vi "运维调试_总氮.vi"() -> ()   [LabVIEW 2016, in "斯坦道总氮.lvlib"]
uses:
  <vilib>/Utility/miscctls.llb/LVPointTypeDef.ctl
  <vilib>/Utility/config.llb/NI_LVConfig.lvlib
  <vilib>/ptbypt/NI_PtbyPt.lvlib
panel:
  in  "模块启用":bool
  in  "串口设置":bool
  in  "备用系数一键写入":bool
  in  "公式一键写入":bool
  in  "流程路径":path=path "C:/Users/STD/Documents/斯坦道流程文件/流程.xml"
  in  "总磷总氮曲线模型":cluster{"X^2":dbl, "X":dbl, "B":dbl}(xcontrol)
  out "字符串 2":string
  in  "质控参数设置":bool
  in  "自动测试量程配置":T1
  out "温度2":sgl
  out "温度1":sgl
  out "ADC":sgl
  out "固件版本号":string
  in  "数组":string[](array[string])
  in  "备用系数写入":bool
  in  "备用系数读取":bool
  in  "备用系数":T2
  in  "量程切换阈值写入":bool
  in  "量程切换阈值读取":bool
  in  "量程切换阈值":cluster{"阈值":dbl, "标液浓度":dbl}
  in  "参数下拉列表":enum16{"总磷", "总氮"}(ring)=enum."总氮"
  in  "量程下拉列表":enum16{"低量程", "高量程"}(ring)
  in  "测量模式下拉列表":enum16{"水样测量", "空白核查", "跨度核查", "标样核查", "加标回收"}(ring)
  in  "公式":cluster{"X^2":dbl, "X":dbl, "b":dbl}
  in  "写公式":bool
  in  "读公式":bool
  in  "返回":bool
  in  "设置":bool
  out "序列号":string="序列号"
  out "测量数据":T3(xcontrol)
  out "集成报警信息":string
  out "定时启动":bool
  out "总磷总氮运行状态":T4(xcontrol)
  in  "停止":bool
  in  "手动启动":bool
  in  "单步测试":bool
  in  "总磷氨氮调试":u16[](xcontrol)
  out "F3":sgl format="%#.6f"
  out "F2":sgl format="%#.6f"
  out "F1":sgl format="%#.6f"
  out "F0":sgl format="%#.6f"
  out "多列列表框":i32(listbox)
  # "参数设置"
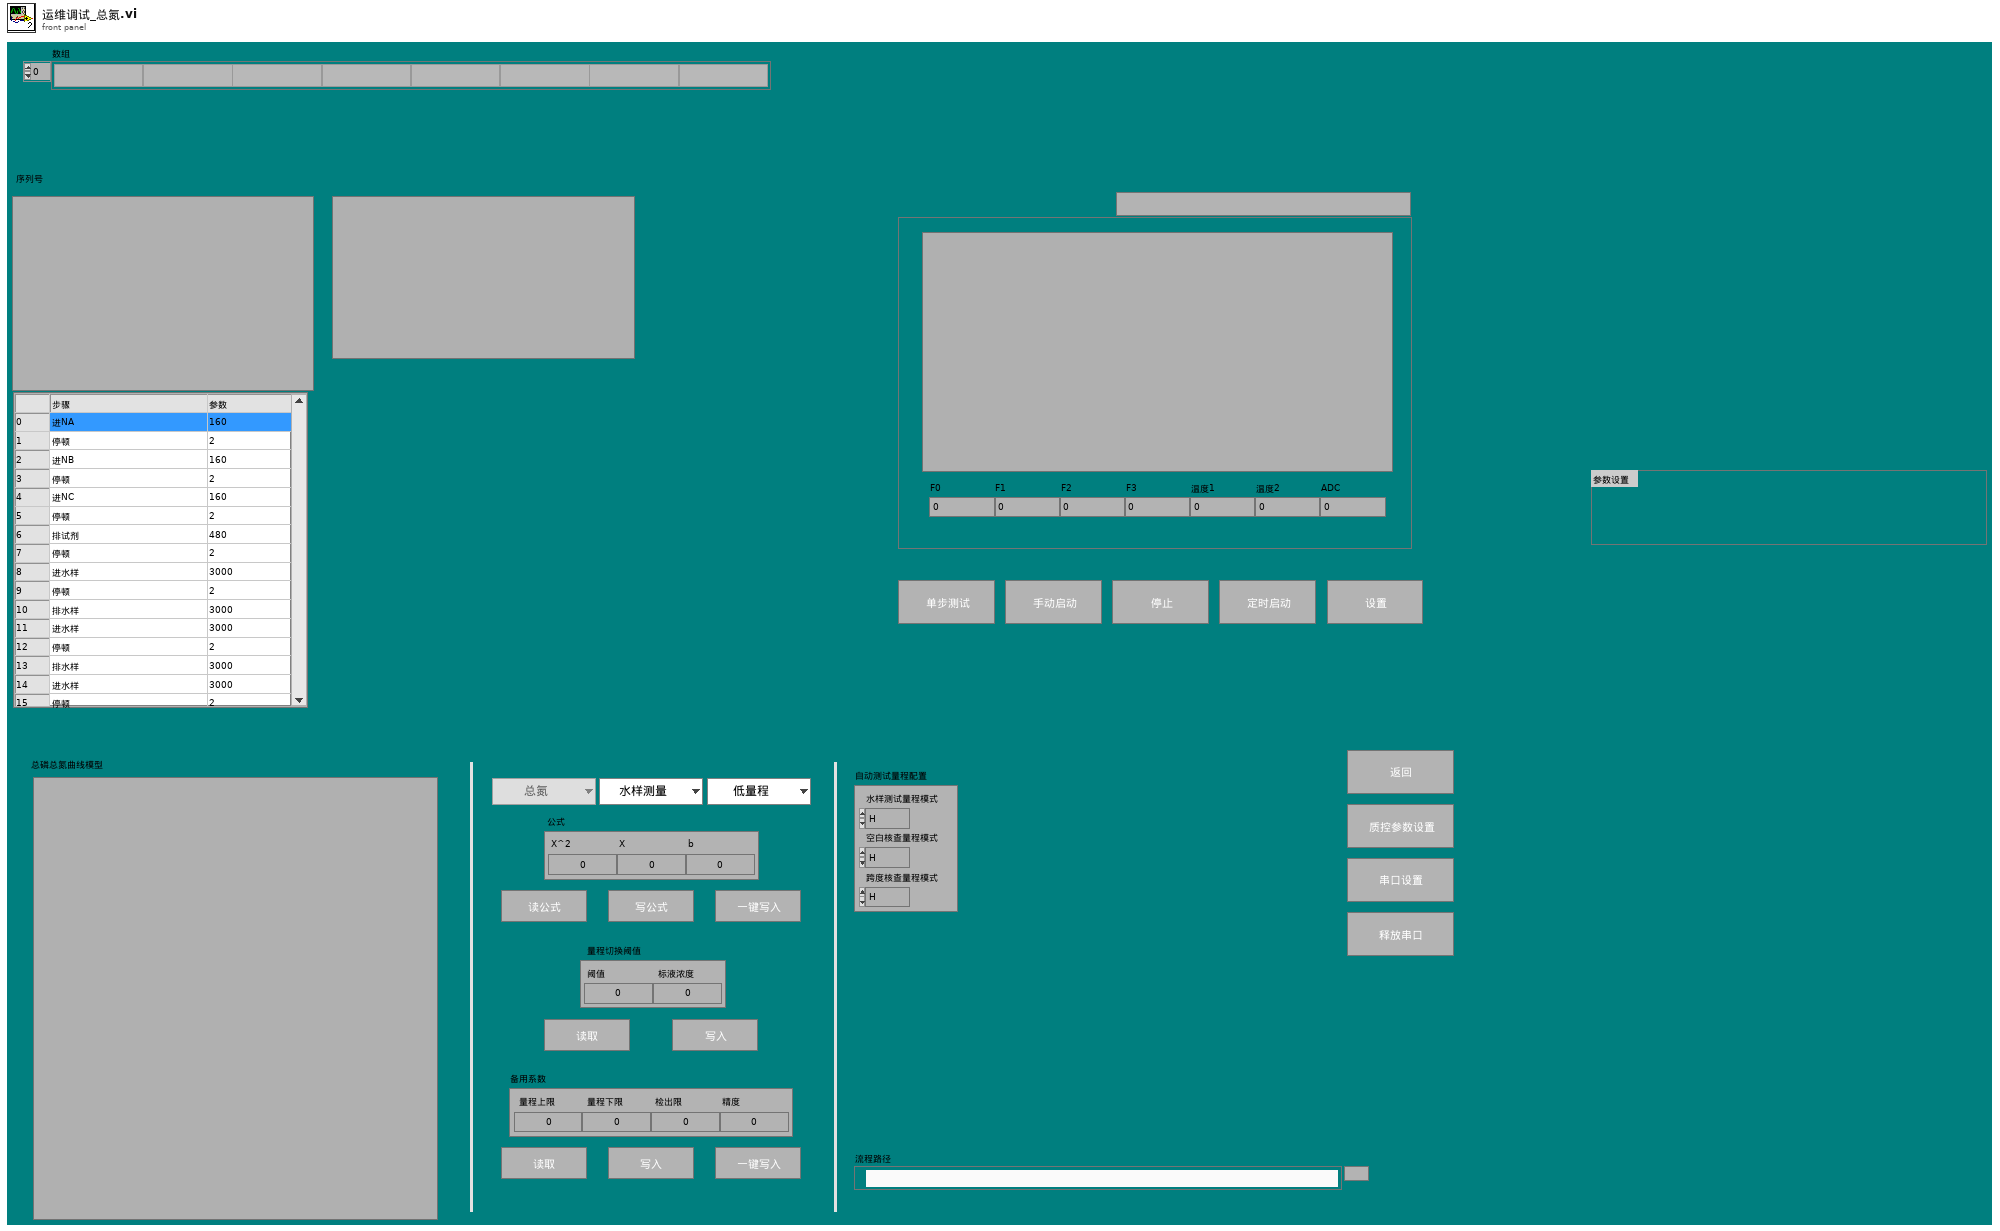
[diagram p1: front panel]
types:
  T1 = cluster{"水样测试量程模式":enum16{"H", "L", "AUTO"}, "空白核查量程模式":enum16{"H", "L", "AUTO"}, "跨度核查量程模式":enum16{"H", "L", "AUTO"}}
  T2 = cluster{"量程上限":dbl, "量程下限":dbl, "检出限":dbl, "精度":dbl}
  T3 = cluster{"flowid":u16, "测量精度":u16, "测量数据区":cluster{"因子编码":u32, "单位":u16, "标样参考值":sgl, "水样数据时间":timestamp, "水样实测值":sgl, "水样数据标识":string, "标样数据时间":timestamp, "标样实测值":sgl, "标样数据标识":string, "空白数据时间":timestamp, "空白实测值":sgl, "空白数据标识":string, "零点核查数据时间":timestamp, "零点核查实测值":sgl, "零点核查数据标识":string, "跨度核查数据时间":timestamp, "跨度核查实测值":sgl, "跨度核查数据标识":string, "加标回收数据时间":timestamp, "加标回收实测值":sgl, "加标回收数据标识":string, "平行样数据时间":timestamp, "平行样实测值":sgl, "平行样数据标识":string, "F0":sgl, "F1":sgl, "F2":sgl, "F3":sgl, "F4":sgl, "F5":sgl, "F6":sgl, "F7":sgl, "温度":sgl, "湿度":sgl, "X值":sgl}}
  T4 = cluster{"系统时间":timestamp, "工作状态":enum16{"空闲", "水样测试", "标样核查", "零点核查", "跨度核查", "空白测试", "平行样测试", "加标回收", "空白校准", "标样校准", "初始化（清洗）"}, "测量模式":enum16{"待机", "连续模式", "周期模式", "定点模式", "受控模式", "手动模式"}, "告警代码":enum16{"无告警", "缺试剂告警", "缺水样告警", "缺蒸馏水告警", "缺标液告警", "仪表漏液告警", "标定异常告警", "超量程告警", "加热异常", "低试剂预警", "超上限告警", "超下限告警", "仪表内部其他异常", "滴定异常告警", "电极异常告警", "量程切换告警", "参数设置告警", "PH电极电位异常", "电导率电极异常", "浊度光度异常", "溶解氧电极异常", "溶解氧光强异常", "温度异常告警", "PH异常告警", "溶解氧异常告警", "电导率异常告警", "浊度异常告警", "叶绿素异常告警", "藻密度异常告警", "蓝绿藻异常告警", "ORP异常告警", "氨氮异常告警", "清洁刷异常告警", "SD卡异常告警", "蓝牙异常告警", "Wifi异常告警", "流程异常告警"}, "故障代码":enum16{"无故障", "电机故障", "温度故障", "通讯故障", "滴定故障"}, "日志代码":u16, "软件版本":u16, "F0":sgl, "F1":sgl, "F2":sgl, "F3":sgl, "T":sgl, "H":sgl, "id":u16, "flowid":u16, "量程":u16, "总磷控温温度1":sgl, "营养盐控温温度2":sgl, "ADC":sgl}
  T5 = cluster{"控制命令":enum16{"启动测量", "标样核查", "零点核查", "跨度核查", "空白测试", "平行样测试", "加标回收", "空白校准", "标样校准", "初始化（清洗）", "停止测试", "仪器重启", "校时", "模式设置", "测量间隔设置"}, "周期设置类型":enum16{"定点启动", "间隔启动"}, "定时功能启用":bool, "定时间隔":dbl, "24H周期设置":bool[]}
  T6 = enum16{"启动测量", "标样核查", "零点核查", "跨度核查", "空白测试", "平行样测试", "加标回收", "空白校准", "标样校准", "初始化（清洗）", "停止测试", "仪器重启", "校时", "模式设置", "测量间隔设置"}
  T7 = enum32{"Bad", "Idle", "Run top level", "Running"}
  T8 = typedef "LVDateTimeRec.ctl" = cluster{"秒数的小数部分":dbl, "秒":i32, "分":i32, "时":i32, "日":i32, "月":i32, "年":i32, "天数（周）":i32, "天数（年）":i32, "DST":i32}
  T9 = typedef "LVPointTypeDef.ctl" = cluster{"Horizontal":i16, "Vertical":i16}
  T10 = cluster{"因子编码":u32, "单位":u16, "标样参考值":sgl, "水样数据时间":timestamp, "水样实测值":sgl, "水样数据标识":string, "标样数据时间":timestamp, "标样实测值":sgl, "标样数据标识":string, "空白数据时间":timestamp, "空白实测值":sgl, "空白数据标识":string, "零点核查数据时间":timestamp, "零点核查实测值":sgl, "零点核查数据标识":string, "跨度核查数据时间":timestamp, "跨度核查实测值":sgl, "跨度核查数据标识":string, "加标回收数据时间":timestamp, "加标回收实测值":sgl, "加标回收数据标识":string, "平行样数据时间":timestamp, "平行样实测值":sgl, "平行样数据标识":string, "F0":sgl, "F1":sgl, "F2":sgl, "F3":sgl, "F4":sgl, "F5":sgl, "F6":sgl, "F7":sgl, "温度":sgl, "湿度":sgl, "X值":sgl}
  T11 = enum16{"空闲", "水样测试", "标样核查", "零点核查", "跨度核查", "空白测试", "平行样测试", "加标回收", "空白校准", "标样校准", "初始化（清洗）"}
  T12 = typedef "NI_LVConfig.lvlib/Config Data RefNum.ctl" = refnum<k1>
  T13 = cluster{"启动模式":enum16{"跨度核查", "水样测量", "空白核查", "标样核查", "加标回收"}, "启动参数":u16, "量程":enum16{"低量程", "高量程"}}
  T14 = cluster{"时间标识":timestamp, "设备":string, "日志信息":string, "流程参数":string}
  T15 = cluster{"时间标识":timestamp, "设备":string, "日志信息":string}
  T16 = enum16{"无告警", "缺试剂告警", "缺水样告警", "缺蒸馏水告警", "缺标液告警", "仪表漏液告警", "标定异常告警", "超量程告警", "加热异常", "低试剂预警", "超上限告警", "超下限告警", "仪表内部其他异常", "滴定异常告警", "电极异常告警", "量程切换告警", "参数设置告警", "PH电极电位异常", "电导率电极异常", "浊度光度异常", "溶解氧电极异常", "溶解氧光强异常", "温度异常告警", "PH异常告警", "溶解氧异常告警", "电导率异常告警", "浊度异常告警", "叶绿素异常告警", "藻密度异常告警", "蓝绿藻异常告警", "ORP异常告警", "氨氮异常告警", "清洁刷异常告警", "SD卡异常告警", "蓝牙异常告警", "Wifi异常告警", "流程异常告警"}
  T17 = typedef "LVRowAndColumnUnsignedTypeDef.ctl" = cluster{"Row":u32, "Column":u32}
  T18 = cluster{"站号":u16, "量程切换":enum32{"H", "L", "AUTO"}, "控制命令":enum16{"启动测量", "标样核查", "零点核查", "跨度核查", "空白测试", "平行样测试", "加标回收", "空白校准", "标样校准", "初始化（清洗）", "停止测试", "仪器重启", "校时", "模式设置", "测量间隔设置"}, "模式设置":enum16{"待机", "连续模式", "周期模式", "定点模式", "受控模式", "手动模式"}, "测量间隔":u16}
  T19 = cluster{"跨度值":dbl, "零点标准液浓度":dbl, "跨度标准液浓度":dbl, "标准液标准浓度":dbl}
  T20 = cluster{"确定":bool, "跨度值":dbl, "零点标准液浓度":dbl, "跨度标准液浓度":dbl, "标准液标准浓度":dbl}
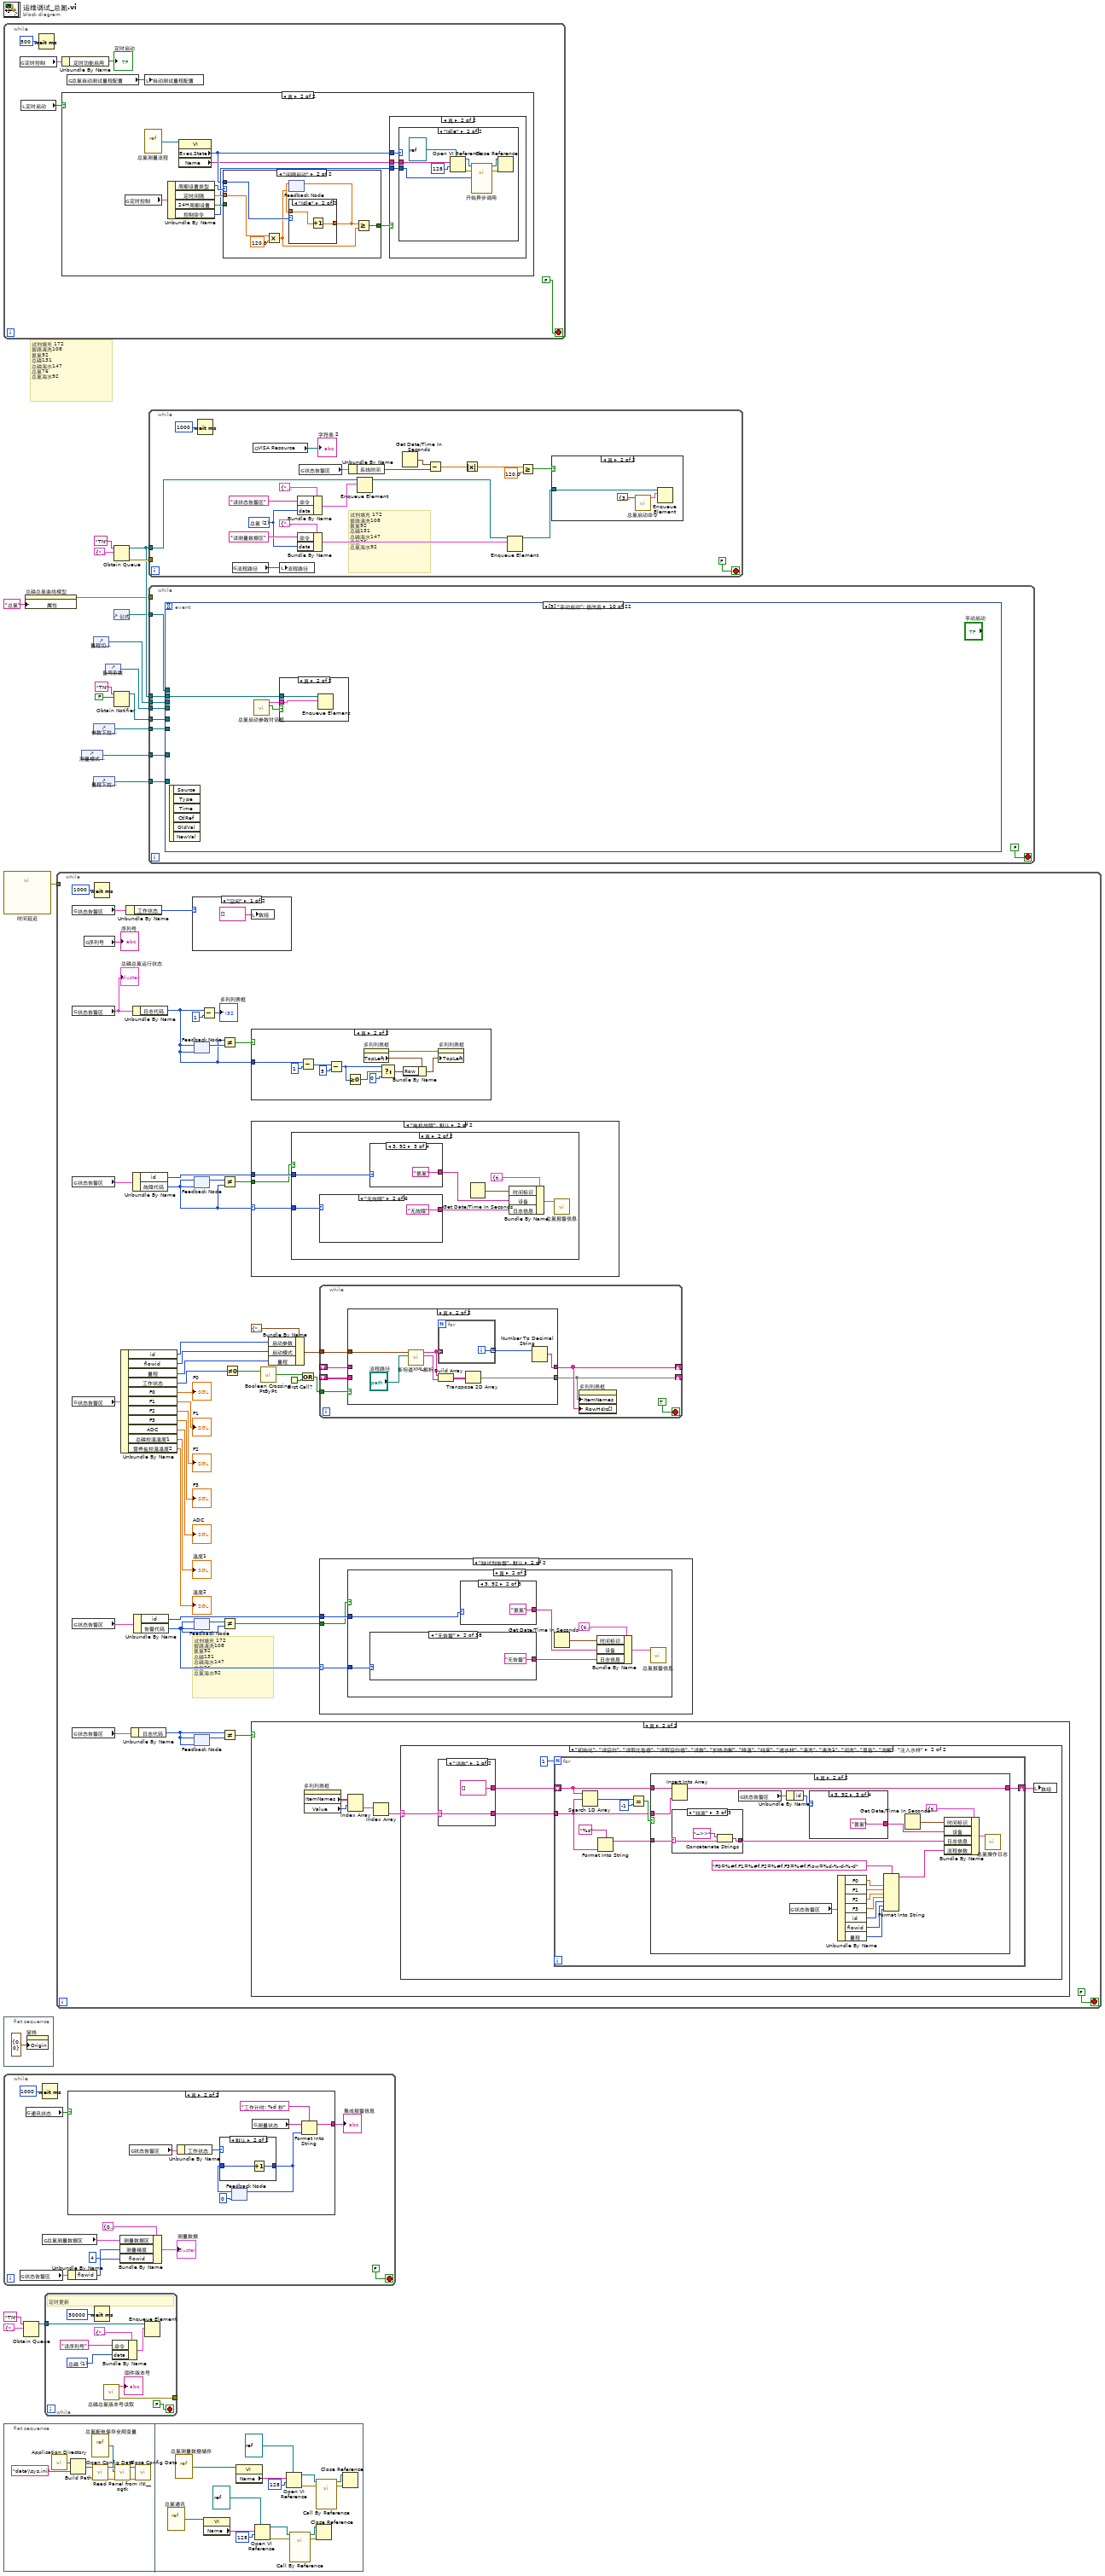
[diagram p0: block diagram]
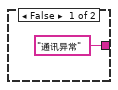
[diagram p2: hidden frame]
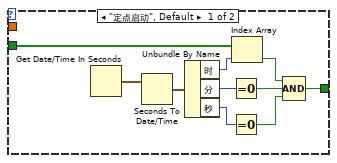
[diagram p7: hidden frame]
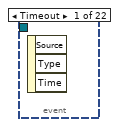
[diagram p9: hidden frame]
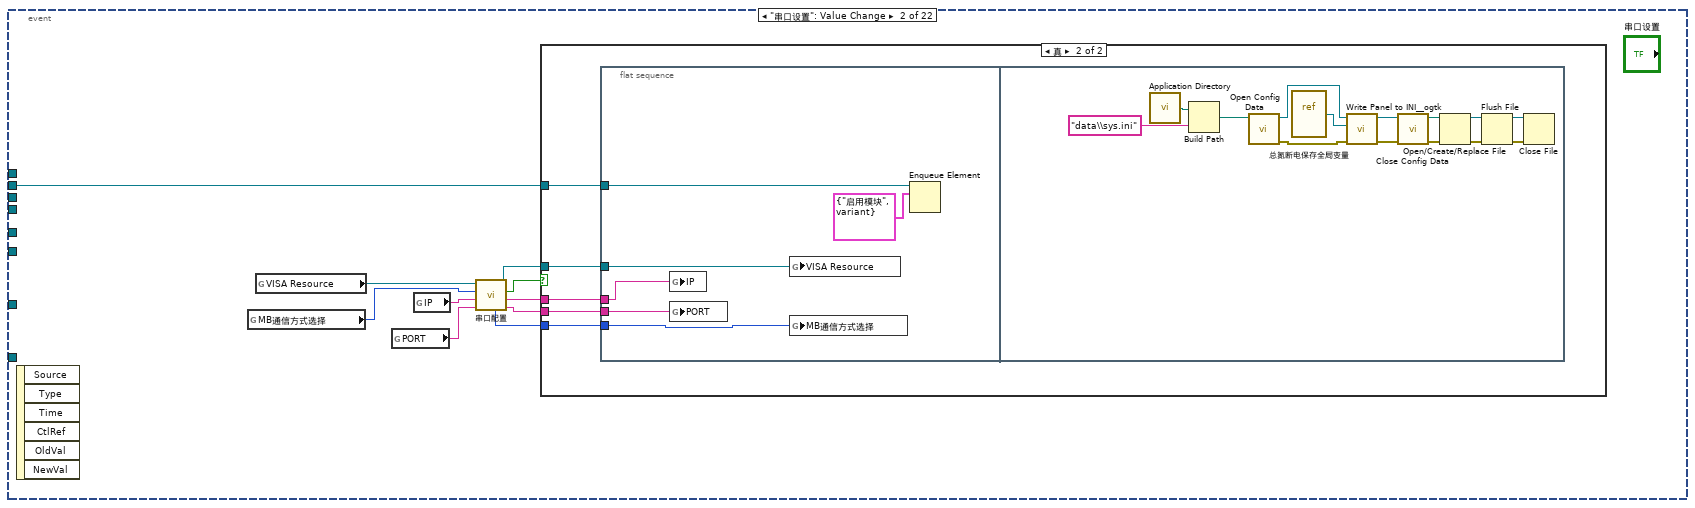
[diagram p10: hidden frame]
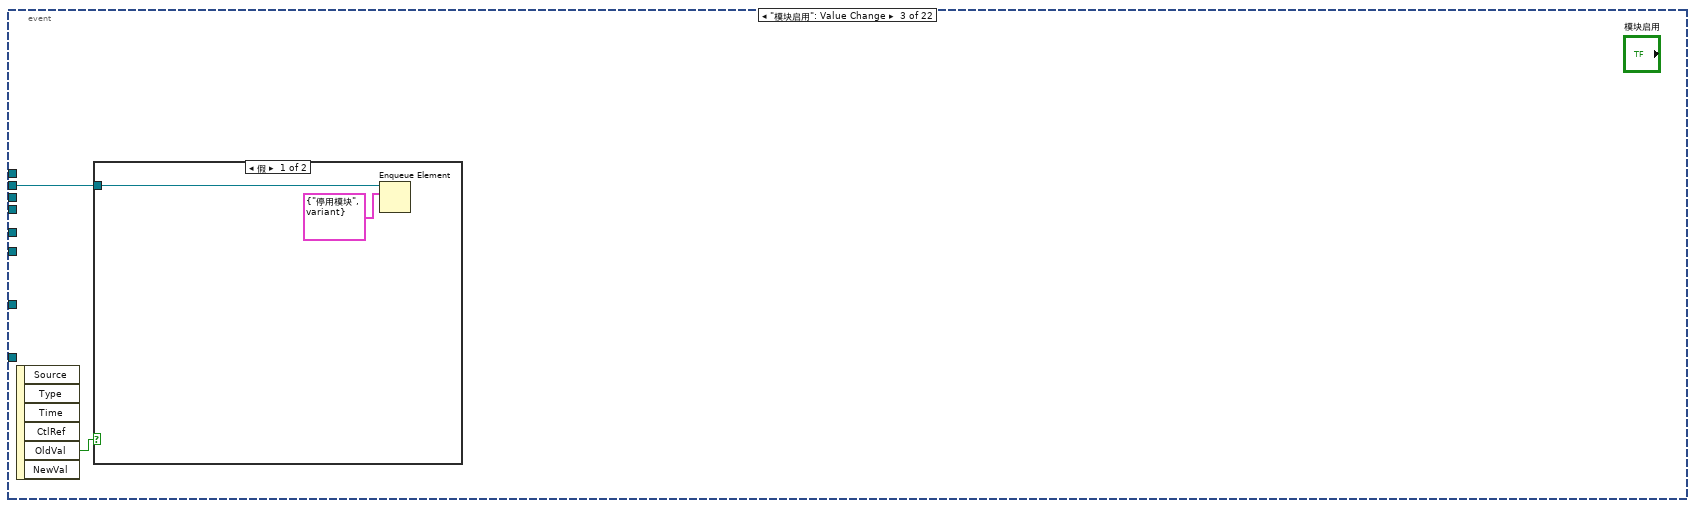
[diagram p12: hidden frame]
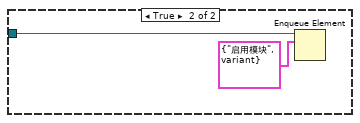
[diagram p13: hidden frame]
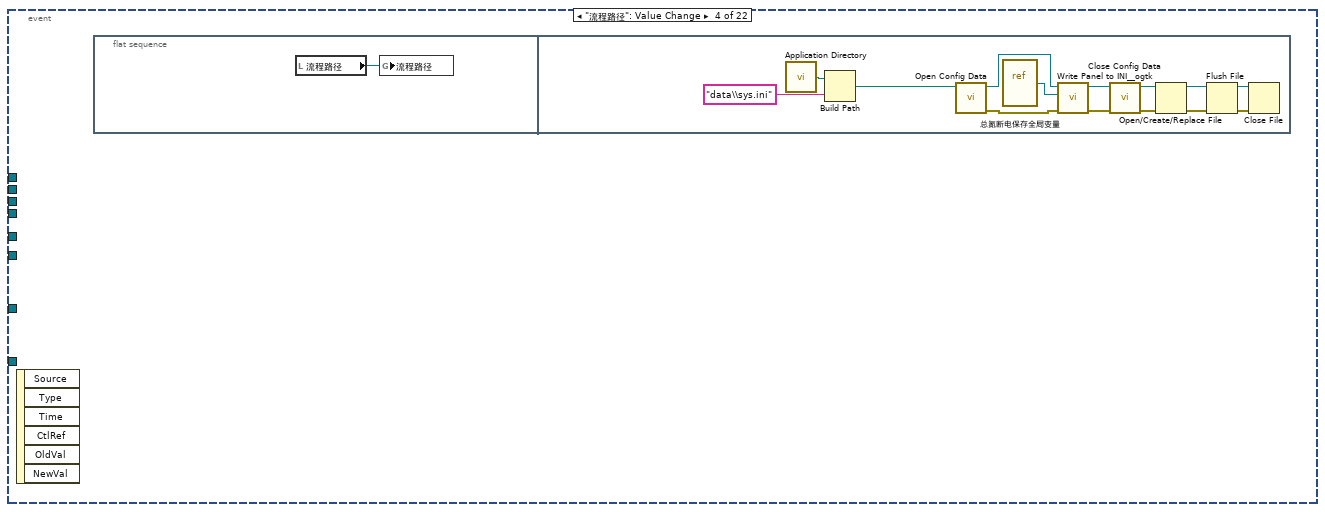
[diagram p14: hidden frame]
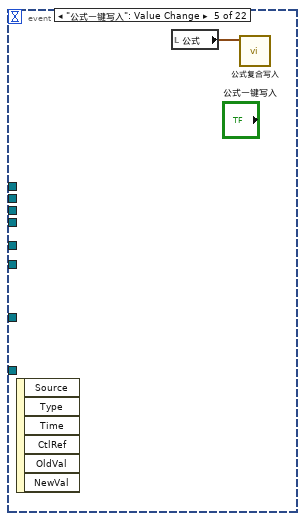
[diagram p15: hidden frame]
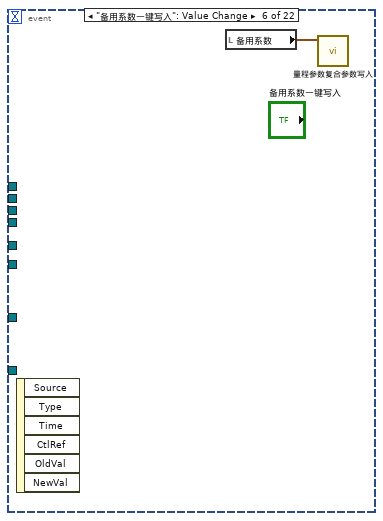
[diagram p16: hidden frame]
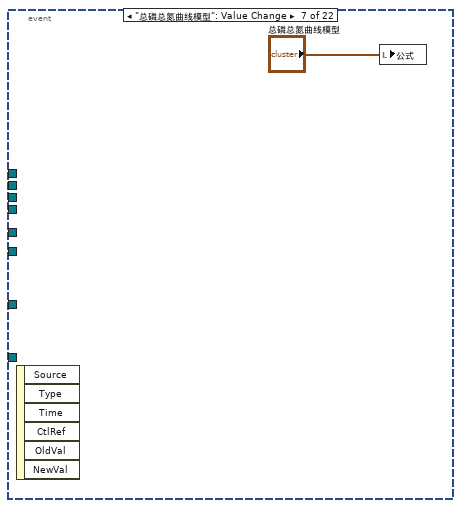
[diagram p17: hidden frame]
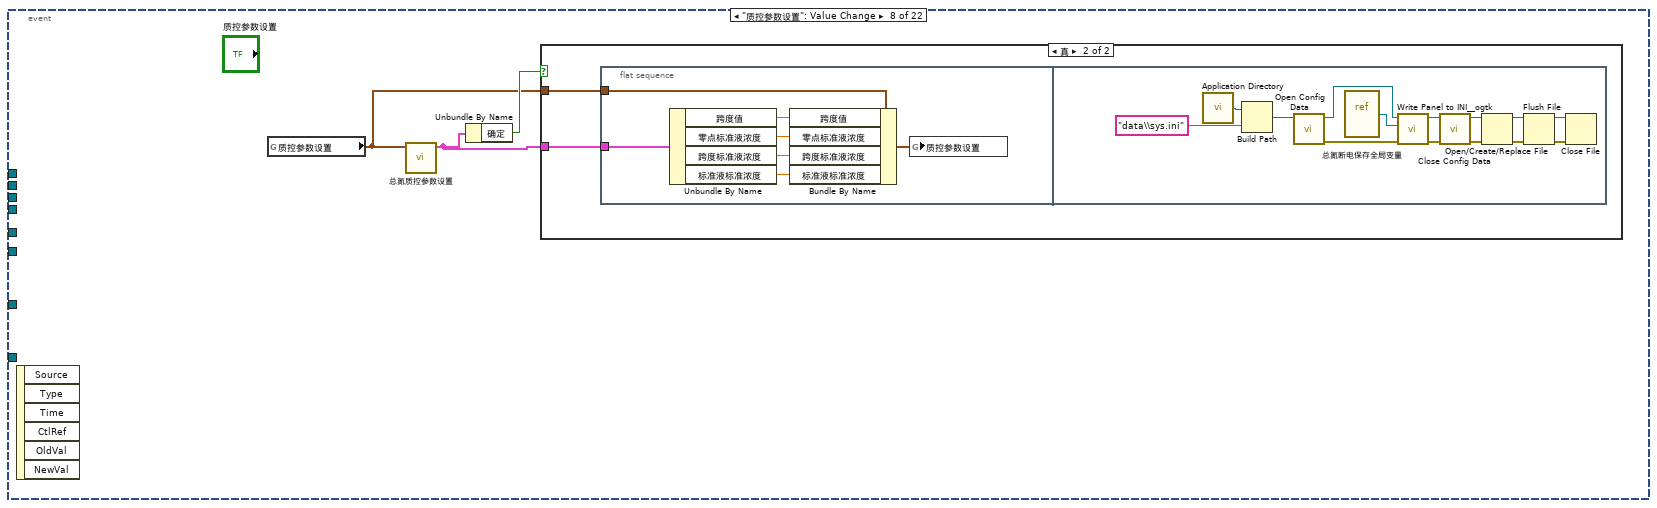
[diagram p18: hidden frame]
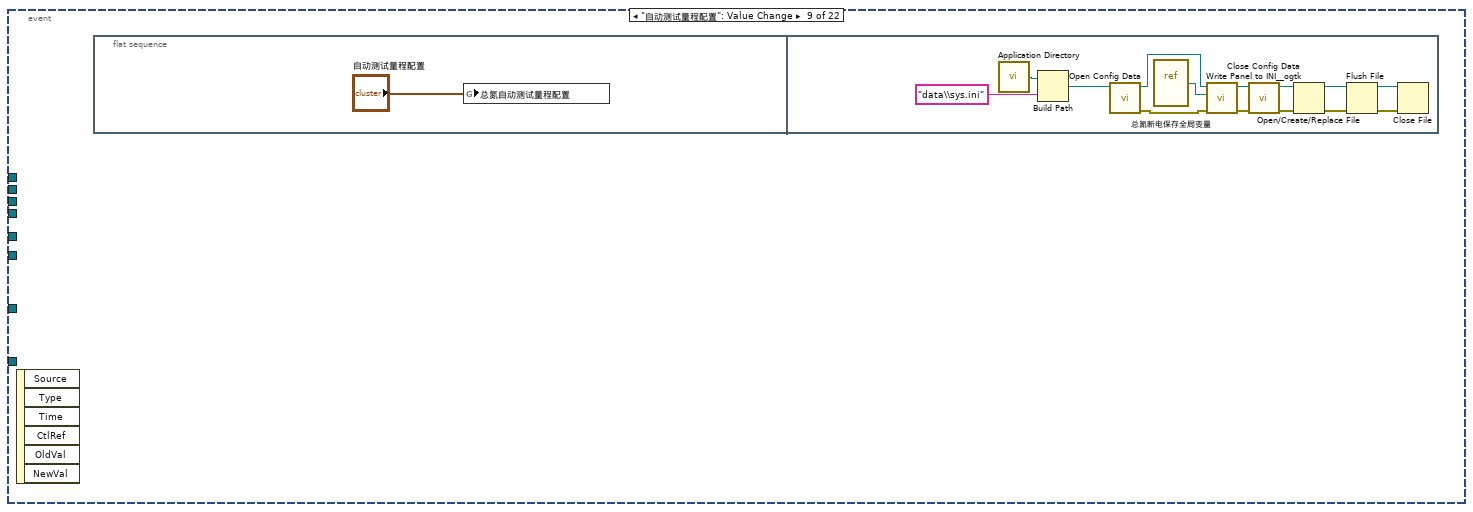
[diagram p20: hidden frame]
diagram:
  # "试剂填充 172 \n管路清洗108\n氨氮92\n总磷131\n总磷海水147\n总氮76\n总氮海水92"
  n1 = while {
    stop <- FALSE stop-if-true
    n2 = global read "总氮断电保存全局变量.vi" "定时控制"() -> (w21:T5)
    n3 = local read "定时启动"() -> (w23:bool)
    n4 = Wait (ms)(milliseconds to wait=u32 500 ("等待时间（毫秒）")) -> ()  [unwired: 1 out]
    n5 = Unbundle By Name(w21) -> ("定时功能启用"=→"定时启动":bool)
    n6 = case shown="真" w23 {
      frame False {
      }
      frame True {
        n7 = global read "总氮断电保存全局变量.vi" "定时控制"() -> (w34:T5)
        n8 = vi-ref "总氮测量流程.vi"() -> (w29:refnum<vi>)
        n9 = Unbundle By Name(w34) -> ("周期设置类型"=w33:enum16{"定点启动", "间隔启动"}, "定时间隔"=w32:dbl, "24H周期设置"=w31:bool[], "控制命令"=w28:T6)
        n10 = property class="VI"(reference=w29) -> ("Exec.State"=w27:T7, "Name"=w26:string)  [unwired: 1 in, 2 out]
        n11 = case shown="\"间隔启动\"" w33 {
          tunnel: w32 -> [_ w59]
          tunnel: w31 -> [w55 _]
          tunnel: w27 -> [_ w62]
          tunnel: [w54 w57] -> w30
          frame "定点启动", Default {
            n12 = Get Date/Time In Seconds() -> (seconds since 1Jan1904=w53:timestamp)
            n13 = Seconds To Date/Time(time stamp (now)=w53) -> (date time rec=w52:T8)  [unwired: 1 in]
            n14 = Unbundle By Name(w52) -> ("时"=w51:i32, "分"=w49:i32, "秒"=w50:i32)
            n15 = Equal To 0?(x=w49) -> (x = 0?=w47:bool)
            n16 = Equal To 0?(x=w50) -> (x = 0?=w46:bool)
            n17 = Index Array(array=w55, index=w51) -> (element=w48:bool)
            n18 = Compound Arithmetic op=AND ("复合运算")(w48, w47, w46) -> (w54:bool)
          }
          frame "间隔启动" {
            n19 = Multiply(x=w59, y=120.0) -> (x*y=w56:dbl)
            n20 = feedback #1(w56) -> (w61:dbl)
            n21 = case shown="\"Idle\"" w62 {
              tunnel: w61 -> [_ w64]
              tunnel: [_ w63] -> w60
              frame "Bad", Default {
              }
              frame "Idle" {
                n22 = Increment(x=w64) -> (x+1=w63:dbl)
              }
            }
            n23 = feedback-in #1(w60) -> ()
            n24 = Greater Or Equal?(x=w60, y=w56) -> (x >= y?=w57:bool)
          }
        }
        n25 = case shown="真" w30 {
          tunnel: w26 -> [_ w37]
          tunnel: w28 -> [_ w36]
          tunnel: w27 -> [_ w35]
          frame False {
          }
          frame True {
            n26 = case shown="\"Idle\"" w35 {
              tunnel: w37 -> [_ w41]
              tunnel: w36 -> [_ w39]
              frame "Bad", Default {
              }
              frame "Idle" {
                n27 = Open VI Reference(type specifier VI Refnum (for type only)=refnum<vi> refnum, vi path=w41, options=128 ("选项")) -> (vi reference=w42:refnum<vi>, error out=w43:errorcluster)  [unwired: 3 in]
                n28 = call-by-ref "开始异步调用"(reference=w42, error in=w43, "控制命令"=w39) -> (reference out=w44:refnum<vi>, error out=w45:errorcluster)  [unwired: 11 in]
                n29 = Close Reference(reference=w44, error in (no error)=w45) -> ()  [unwired: 1 out]
              }
            }
          }
        }
      }
    }
    n30 = global read "总氮断电保存全局变量.vi" "总氮自动测试量程配置"() -> (w22:T1)
    n31 = local write "自动测试量程配置"(w22) -> ()
  }
  n32 = call "时间延迟"() -> ("error out"=w9:errorcluster)  [unwired: 11 in]
  n33 = flat-sequence {
    frame #0 {
      n34 = property on="窗格" class="Pane"("Origin"=T9 {"Horizontal"=0, "Vertical"=0} ("原点")) -> ()  [unwired: 2 in, 2 out]
    }
  }
  n35 = while {
    stop <- FALSE stop-if-true
    n36 = global read "VAR总氮全局变量.vi" "状态告警区"() -> (w71:T4)
    n37 = global read "VAR总氮全局变量.vi" "通讯状态"() -> (w73:bool)
    n38 = Wait (ms)(milliseconds to wait=u32 1000 ("等待时间（毫秒）")) -> ()  [unwired: 1 out]
    n39 = global read "VAR总氮全局变量.vi" "总氮测量数据区"() -> (w66:T10)
    n40 = case shown="真" w73 {
      tunnel: ["通讯异常" ("集成报警信息") w78] -> w72
      frame False {
      }
      frame True {
        n41 = global read "VAR总氮全局变量.vi" "状态告警区"() -> (w84:T4)
        n42 = Unbundle By Name(w84) -> ("工作状态"=w83:T11)
        n43 = feedback #2(0) -> (w81:i32)
        n44 = case shown="默认" w83 {
          tunnel: w81 -> [_ w86]
          tunnel: [_ w85] -> w79
          frame "空闲" {
          }
          frame Default {
            n45 = Increment(x=w86) -> (x+1=w85:i32)
          }
        }
        n46 = feedback-in #2(w79) -> ()
        n47 = global read "VAR总氮全局变量.vi" "测量状态"() -> (w77:string)
        n48 = Format Into String(format string="工作计时: %d 秒" ("格式字符串"), initial string=w77, w79) -> (resulting string=w78:string)  [unwired: 1 in, 1 out]
      }
    }
    "集成报警信息" <- w72
    n49 = Unbundle By Name(w71) -> ("flowid"=w70:u16)
    n50 = Bundle By Name(cluster=T3 {"flowid"=0, "测量精度"=0, "测量数据区"={"因子编码"=0, "单位"=0, "标样参考值"=0.0, "水样数据时间"=timestamp(0 s since 1904-01-01), "水样实测值"=0.0, "水样数据标识"="", "标样数据时间"=timestamp(0 s since 1904-01-01), "标样实测值"=0.0, "标样数据标识"="", "空白数据时间"=timestamp(0 s since 1904-01-01), "空白实测值"=0.0, "空白数据标识"="", "零点核查数据时间"=timestamp(0 s since 1904-01-01), "零点核查实测值"=0.0, "零点核查数据标识"="", "跨度核查数据时间"=timestamp(0 s since 1904-01-01), "跨度核查实测值"=0.0, "跨度核查数据标识"="", "加标回收数据时间"=timestamp(0 s since 1904-01-01), "加标回收实测值"=0.0, "加标回收数据标识"="", "平行样数据时间"=timestamp(0 s since 1904-01-01), "平行样实测值"=0.0, "平行样数据标识"="", "F0"=0.0, "F1"=0.0, "F2"=0.0, "F3"=0.0, "F4"=0.0, "F5"=0.0, "F6"=0.0, "F7"=0.0, "温度"=0.0, "湿度"=0.0, "X值"=0.0}} ("总氮测量数据"), "测量数据区"=w66, "测量精度"=u16 4, "flowid"=w70) -> (→"测量数据":T3)
  }
  n51 = flat-sequence {
    frame #0 {
      n52 = call <vilib>:"Application Directory.vi"() -> ("Application Directory"=w94:path)
      n53 = Build Path(base path=w94, name or relative path="data\\sys.ini" ("名称或相对路径")) -> (appended path=w92:path)
      n54 = vi-ref "总氮断电保存全局变量.vi"() -> (w90:refnum<vi>)
      n55 = call <vilib>:"Open Config Data.vi"("configuration file path"=w92) -> ("error out"=w88:errorcluster, "refnum"=w91:T12)  [unwired: 8 in, 1 out]
      n56 = call <userlib>:"Read Panel from INI__ogtk.vi"("error in (no error)"=w88, "VI ref"=w90, "refnum"=w91) -> ("error out"=w87:errorcluster, "refnum out"=w89:T12)  [unwired: 7 in]
      n57 = call <vilib>:"Close Config Data.vi"("error in (no error)"=w87, "refnum"=w89) -> ()  [unwired: 8 in, 2 out]
    }
    frame #1 {
      n58 = vi-ref "总氮通讯.vi"() -> (w110:refnum<vi>)
      n59 = vi-ref "总氮测量数据储存.vi"() -> (w102:refnum<vi>)
      n60 = property class="VI"(reference=w110) -> ("Name"=w109:string)  [unwired: 1 in, 2 out]
      n61 = property class="VI"(reference=w102) -> ("Name"=w95:string)  [unwired: 1 in, 2 out]
      n62 = Open VI Reference(type specifier VI Refnum (for type only)=refnum<vi> refnum, vi path=w109, options=128 ("选项")) -> (vi reference=w107:refnum<vi>, error out=w105:errorcluster)  [unwired: 3 in]
      n63 = Open VI Reference(type specifier VI Refnum (for type only)=refnum<vi> refnum, vi path=w95, options=128 ("选项")) -> (vi reference=w97:refnum<vi>, error out=w99:errorcluster)  [unwired: 3 in]
      n64 = call-by-ref "?"(reference=w107, error in=w105) -> (reference out=w103:refnum<vi>, error out=w104:errorcluster)  [unwired: 12 in]
      n65 = call-by-ref "?"(reference=w97, error in=w99) -> (reference out=w101:refnum<vi>, error out=w100:errorcluster)  [unwired: 12 in]
      n66 = Close Reference(reference=w103, error in (no error)=w104) -> ()  [unwired: 1 out]
      n67 = Close Reference(reference=w101, error in (no error)=w100) -> ()  [unwired: 1 out]
    }
  }
  n68 = Obtain Queue(name (unnamed)="TN" ("名称（未命名）"), element data type=cluster{"命令":string, "data":variant} {"命令"="", "data"=variant}) -> (queue out=w6:refnum<queue>)  [unwired: 3 in, 2 out]
  n69 = property on="总磷总氮曲线模型" class="曲线模型 (严格)"("属性"="总氮" ("调用模块名称属性")) -> (error out=w4:errorcluster)  [unwired: 2 in, 1 out]
  n70 = while {
    tunnel: w6 -> [w115]
    tunnel: [w111] -> _
    stop <- FALSE stop-if-true
    w116 = u16 1 items=["总磷"=1, "氨氮"=3] ("站号")
    # "定时更新"
    n71 = Wait (ms)(milliseconds to wait=u32 30000 ("等待时间（毫秒）")) -> ()  [unwired: 1 out]
    n72 = call "总磷总氮版本号读取.vi"() -> ("error out"=w111:errorcluster, "固件版本号"=→"固件版本号":string)  [unwired: 10 in]
    n73 = Bundle By Name(cluster=cluster{"命令":string, "data":variant} {"命令"="", "data"=variant} ("元素"), "命令"="读序列号", "data"=w116) -> (w114:cluster{"命令":string, "data":variant})
    n74 = Enqueue Element(queue=w115, element=w114) -> ()  [unwired: 2 in, 3 out]
  }
  n75 = while {
    tunnel: w9 -> [_]
    stop <- FALSE stop-if-true
    # "试剂填充 172 \n管路清洗108\n氨氮92\n总磷131\n总磷海水147\n总氮76\n总氮海水92"
    n76 = global read "VAR总氮全局变量.vi" "状态告警区"() -> (w134:T4)
    n77 = global read "VAR总氮全局变量.vi" "状态告警区"() -> (w147:T4)
    "总磷总氮运行状态" <- w147
    n78 = global read "VAR总氮全局变量.vi" "状态告警区"() -> (w139:T4)
    n79 = global read "VAR总氮全局变量.vi" "状态告警区"() -> (w155:T4)
    n80 = global read "VAR总氮全局变量.vi" "状态告警区"() -> (w144:T4)
    n81 = global read "VAR总氮全局变量.vi" "状态告警区"() -> (w131:T4)
    n82 = global read "VAR总氮全局变量.vi" "序列号"() -> (→"序列号":string)
    n83 = Wait (ms)(milliseconds to wait=u32 1000 ("等待时间（毫秒）")) -> ()  [unwired: 1 out]
    n84 = Unbundle By Name(w155) -> ("id"=w152:u16, "flowid"=w154:u16, "量程"=w153:u16, "工作状态"=w121:T11, "F0"=→"F0":sgl, "F1"=→"F1":sgl, "F2"=→"F2":sgl, "F3"=→"F3":sgl, "ADC"=→"ADC":sgl, "总磷控温温度1"=→"温度1":sgl, "营养盐控温温度2"=→"温度2":sgl)
    n85 = Unbundle By Name(w134) -> ("工作状态"=w133:T11)
    n86 = Unbundle By Name(w131) -> ("日志代码"=w130:u16)
    n87 = Unbundle By Name(w147) -> ("日志代码"=w127:u16)
    n88 = Unbundle By Name(w139) -> ("id"=w138:u16, "故障代码"=w135:enum16{"无故障", "电机故障", "温度故障", "通讯故障", "滴定故障"})
    n89 = Unbundle By Name(w144) -> ("id"=w143:u16, "告警代码"=w140:T16)
    n90 = case shown="\"空闲\"" w133 {
      frame "空闲" {
        n91 = local write "数组"(string[] [] ("数组")) -> ()
      }
      frame "水样测试", Default {
      }
    }
    n92 = feedback-in #3(w127) -> ()
    n93 = feedback #3(w127) -> (w160:u16)
    n94 = feedback #4(w135) -> (w136:enum16{"无故障", "电机故障", "温度故障", "通讯故障", "滴定故障"})
    n95 = feedback-in #4(w135) -> ()
    n96 = feedback #5(w140) -> (w141:T16)
    n97 = feedback-in #5(w140) -> ()
    n98 = feedback #6(w130) -> (w132:u16)
    n99 = feedback-in #6(w130) -> ()
    n100 = Subtract(x=w127, y=1) -> (x-y=→"多列列表框":i32)
    n101 = Not Equal?(x=w127, y=w160) -> (x != y?=w159:bool)
    n102 = Not Equal?(x=w136, y=w135) -> (x != y?=w137:bool)
    n103 = Not Equal?(x=w141, y=w140) -> (x != y?=w142:bool)
    n104 = Not Equal?(x=w130, y=w132) -> (x != y?=w129:bool)
    n105 = Not Equal To 0?(x=w121) -> (x != 0?=w157:bool)
    n106 = case shown="真" w159 {
      tunnel: w127 -> [_ w313]
      frame False {
      }
      frame True {
        n107 = Subtract(x=w313, y=1) -> (x-y=w311:i32)
        n108 = Subtract(x=w311, y=5) -> (x-y=w315:i32)
        n109 = Greater Or Equal To 0?(x=w315) -> (x >= 0?=w314:bool)
        n110 = property on="多列列表框" class="MCListbox (严格)"() -> (error out=w319:errorcluster, "TopLeft"=w320:T17)  [unwired: 2 in, 1 out]
        n111 = Select(t=w315, s=w314, f=0) -> (s? t:f=w316:i32)
        n112 = Bundle By Name(cluster=w320, "Row"=w316) -> (w321:T17)
        n113 = property on="多列列表框" class="MCListbox (严格)"(error in=w319, "TopLeft"=w321) -> ()  [unwired: 1 in, 2 out]
      }
    }
    n114 = case shown="\"电机故障\", 默认" w135 {
      selector: w135 -> [_ w218]
      tunnel: w138 -> [_ w219]
      tunnel: w137 -> [_ w217]
      frame "无故障" {
      }
      frame "电机故障", Default {
        n115 = case shown="真" w217 {
          tunnel: w219 -> [_ w226]
          tunnel: w218 -> [_ w221]
          frame False {
          }
          frame True {
            n116 = case shown="\"无故障\"" w221 {
              selector: w221 -> [w228 _ _ _ _ _]
              tunnel: [w227 "无故障" "电机故障" "温度故障" "通讯故障" "滴定故障"] -> w220
              frame Default {
                n117 = Format Into String(format string="%d" ("格式字符串"), initial string="未知" ("工作状态"), w228) -> (resulting string=w227:string)  [unwired: 1 in, 1 out]
              }
              frame "无故障" {
              }
              frame "电机故障" {
              }
              frame "温度故障" {
              }
              frame "通讯故障" {
              }
              frame "滴定故障" {
              }
            }
            n118 = case shown="3, 92" w226 {
              tunnel: [_ "总磷" ("table输入") "氨氮" ("table输入") "总氮" ("table输入")] -> w222
              frame Default {
              }
              frame 1, 131 {
              }
              frame 3, 92 {
              }
              frame 2, 76 {
              }
            }
            n119 = Get Date/Time In Seconds() -> (seconds since 1Jan1904=w223:timestamp)
            n120 = Bundle By Name(cluster=T15 {"时间标识"=timestamp(0 s since 1904-01-01), "设备"="", "日志信息"=""} ("data in"), "时间标识"=w223, "设备"=w222, "日志信息"=w220) -> (w224:T15)
            n121 = call "总氮报警信息.vi"("data in"=w224) -> ()  [unwired: 11 in]
          }
        }
      }
    }
    n122 = case shown="真" w129 {
      frame False {
      }
      frame True {
        n123 = property on="多列列表框" class="MCListbox (严格)"() -> ("ItemNames"=w166:string[][], "Value"=w167:i32)  [unwired: 2 in, 2 out]
        n124 = Index Array(array=w166, index (row)=w167) -> (element=w165:string[])  [unwired: 1 in]
        n125 = Index Array(array=w165) -> (element=w164:string)  [unwired: 1 in]
        n126 = case shown="\"初始化\", \"读空白\", \"读取比色值\", \"读取空白值\", \"读数\", \"加热消解\", \"降温\", \"结束\", \"进水样\", \"清洗\", \"清洗1\", \"润洗\", \"显色\", \"消解\", \"注入水样\"" w164 {
          selector: w164 -> [_ w170]
          frame Default {
          }
          frame "初始化", "读空白", "读取比色值", "读取空白值", "读数", "加热消解", "降温", "结束", "进水样", "清洗", "清洗1", "润洗", "显色", "消解", "注入水样" {
            n127 = case shown="\"读数\"" w170 {
              selector: w170 -> [w174 w176]
              tunnel: [w174 w176] -> w169
              tunnel: [string[] [] ("数组") "数组"] -> w168
              frame "读数" {
              }
              frame Default {
              }
            }
            n128 = for {
              N: 1 -> [_]
              tunnel: w169 -> [w178]
              shift-right: [w177] -> w171
              shift-left: w168 -> [w179]
              n129 = Search 1D Array(1D array=w179, element=w178) -> (index of element=w182:i32)  [unwired: 1 in]
              n130 = Format Into String(format string="%s" ("格式字符串"), w178) -> (resulting string=w183:string)  [unwired: 2 in, 1 out]
              n131 = Equal?(x=w182, y=-1) -> (x = y?=w180:bool)
              n132 = case shown="真" w180 {
                tunnel: w183 -> [_ w187]
                tunnel: w179 -> [w185 w191]
                tunnel: w178 -> [_ w190]
                tunnel: [w185 w189] -> w177
                frame False {
                }
                frame True {
                  n133 = Insert Into Array(array=w191, new element=w190) -> (w189:string[])  [unwired: 1 in]
                  n134 = case shown="\"结束\"" w187 {
                    selector: w187 -> [w207 w210 w213]
                    tunnel: [w207 w209 w212] -> w186
                    frame Default {
                    }
                    frame "初始化" {
                      n135 = Concatenate Strings("-->>" ("字符串"), w210) -> (w209:string)
                    }
                    frame "结束" {
                      n136 = Concatenate Strings("-->>" ("字符串"), w213) -> (w212:string)
                    }
                  }
                  n137 = global read "VAR总氮全局变量.vi" "状态告警区"() -> (w206:T4)
                  n138 = Unbundle By Name(w206) -> ("id"=w205:u16)
                  n139 = global read "VAR总氮全局变量.vi" "状态告警区"() -> (w201:T4)
                  n140 = case shown="3, 92" w205 {
                    tunnel: [_ "总磷" ("table输入") "氨氮" ("table输入") "总氮" ("table输入")] -> w203
                    frame Default {
                    }
                    frame 1, 131 {
                    }
                    frame 3, 92 {
                    }
                    frame 2, 76 {
                    }
                  }
                  n141 = Unbundle By Name(w201) -> ("F0"=w198:sgl, "F1"=w197:sgl, "F2"=w196:sgl, "F3"=w195:sgl, "id"=w194:u16, "flowid"=w193:u16, "量程"=w192:u16)
                  n142 = Format Into String(format string="F0=%#f,F1=%#f,F2=%#f,F3=%#f,Flow=%d-%-d-%-d" ("格式字符串"), w198, w197, w196, w195, w194, w193, w192) -> (resulting string=w199:string)  [unwired: 2 in, 1 out]
                  n143 = Get Date/Time In Seconds() -> (seconds since 1Jan1904=w202:timestamp)
                  n144 = Bundle By Name(cluster=T14 {"时间标识"=timestamp(0 s since 1904-01-01), "设备"="", "日志信息"="", "流程参数"=""} ("data in"), "时间标识"=w202, "设备"=w203, "日志信息"=w186, "流程参数"=w199) -> (w204:T14)
                  n145 = call "总氮操作日志.vi"("data in"=w204) -> ()  [unwired: 11 in]
                }
              }
            }
            n146 = local write "数组"(w171) -> ()
          }
        }
      }
    }
    n147 = call <vilib>:"Boolean Crossing PtByPt.vi"("input"=w157) -> ("crossing"=w120:bool)  [unwired: 2 in]
    n148 = Bundle By Name(cluster=T13 {"启动模式"=enum."跨度核查", "启动参数"=1, "量程"=enum."低量程"} ("参数簇"), "启动参数"=w152, "启动模式"=w154, "量程"=w153) -> (w146:T13)
    n149 = First Call?() -> (First Call?: T/F=w158:bool)
    n150 = Or(x=w120, y=w158) -> (x .or. y?=w156:bool)
    n151 = while {
      tunnel: w156 -> [w299]
      tunnel: w146 -> [w298]
      shift-right: [w293] -> _
      shift-left: _ -> [w295]
      shift-right: [w294] -> _
      shift-left: _ -> [w296]
      stop <- TRUE stop-if-true
      n152 = case shown="真" w299 {
        tunnel: [w301 w309] -> w294
        tunnel: [w300 w308] -> w293
        tunnel: w298 -> [_ w303]
        tunnel: w296 -> [w301 _]
        tunnel: w295 -> [w300 _]
        frame False {
        }
        frame True {
          n153 = call "斯坦道XML解析.vi"("添加的路径"="流程路径", "参数簇"=w303) -> ("步骤时间"=w304:string[], "步骤名"=w306:string[])  [unwired: 8 in]
          n154 = for {
            tunnel: w306 -> [_] mode=indexing
            tunnel: [w310] -> w307 mode=indexing
            i -> [w310]
          }
          n155 = Build Array(w306, w304) -> (w305:string[][])
          n156 = Transpose 2D Array(2D array=w305) -> (transposed array=w308:string[][])
          n157 = Number To Decimal String(number=w307) -> (decimal integer string=w309:string[])  [unwired: 1 in]
        }
      }
      n158 = property on="多列列表框" class="MCListbox (严格)"("ItemNames"=w293, "RowHdrs[]"=w294) -> ()  [unwired: 2 in, 2 out]
    }
    n159 = case shown="\"缺试剂告警\", 默认" w140 {
      selector: w140 -> [_ w240]
      tunnel: w143 -> [_ w241]
      tunnel: w142 -> [_ w239]
      frame "无告警" {
      }
      frame "缺试剂告警", Default {
        n160 = case shown="真" w239 {
          tunnel: w241 -> [_ w248]
          tunnel: w240 -> [_ w242]
          frame False {
          }
          frame True {
            n161 = case shown="\"无告警\"" w242 {
              selector: w242 -> [w250 _ _ _ _ _ _ _ _ _ _ _ _ _ _ _ _ _ _ _ _ _ _ _ _ _ _ _ _ _ _ _ _ _ _ _ _ _]
              tunnel: [w249 "无告警" "缺试剂告警" "缺水样告警" "缺蒸馏水告警" "缺标液告警" "仪表漏液告警" "标定异常告警" "超量程告警" "加热异常" "低试剂预警" "超上限告警" "超下限告警" "仪表内部其他异常" "滴定异常告警" "电极异常告警" "量程切换告警" "参数设置告警" "PH电极电位异常" "电导率电极异常" "浊度光度异常" "溶解氧电极异常" "溶解氧光强异常" "温度异常告警" "PH异常告警" "溶解氧异常告警" "电导率异常告警" "浊度异常告警" "叶绿素异常告警" "藻密度异常告警" "蓝绿藻异常告警" "ORP异常告警" "氨氮异常告警" "清洁刷异常告警" "SD卡异常告警" "蓝牙异常告警" "WiFi异常告警" "流程异常告警"] -> w243
              frame Default {
                n162 = Format Into String(format string="%d" ("格式字符串"), initial string="未知" ("工作状态"), w250) -> (resulting string=w249:string)  [unwired: 1 in, 1 out]
              }
              frame "无告警" {
              }
              frame "缺试剂告警" {
              }
              frame "缺水样告警" {
              }
              frame "缺蒸馏水告警" {
              }
              frame "缺标液告警" {
              }
              frame "仪表漏液告警" {
              }
              frame "标定异常告警" {
              }
              frame "超量程告警" {
              }
              frame "加热异常" {
              }
              frame "低试剂预警" {
              }
              frame "超上限告警" {
              }
              frame "超下限告警" {
              }
              frame "仪表内部其他异常" {
              }
              frame "滴定异常告警" {
              }
              frame "电极异常告警" {
              }
              frame "量程切换告警" {
              }
              frame "参数设置告警" {
              }
              frame "PH电极电位异常" {
              }
              frame "电导率电极异常" {
              }
              frame "浊度光度异常" {
              }
              frame "溶解氧电极异常" {
              }
              frame "溶解氧光强异常" {
              }
              frame "温度异常告警" {
              }
              frame "PH异常告警" {
              }
              frame "溶解氧异常告警" {
              }
              frame "电导率异常告警" {
              }
              frame "浊度异常告警" {
              }
              frame "叶绿素异常告警" {
              }
              frame "藻密度异常告警" {
              }
              frame "蓝绿藻异常告警" {
              }
              frame "ORP异常告警" {
              }
              frame "氨氮异常告警" {
              }
              frame "清洁刷异常告警" {
              }
              frame "SD卡异常告警" {
              }
              frame "蓝牙异常告警" {
              }
              frame "Wifi异常告警" {
              }
              frame "流程异常告警" {
              }
            }
            n163 = case shown="3, 92" w248 {
              tunnel: ["总磷" ("table输入") "氨氮" ("table输入") "总氮" ("table输入")] -> w244
              frame 1, 131 {
              }
              frame 3, 92 {
              }
              frame 2, 76, Default {
              }
            }
            n164 = Get Date/Time In Seconds() -> (seconds since 1Jan1904=w245:timestamp)
            n165 = Bundle By Name(cluster=T15 {"时间标识"=timestamp(0 s since 1904-01-01), "设备"="", "日志信息"=""} ("data in"), "时间标识"=w245, "设备"=w244, "日志信息"=w243) -> (w246:T15)
            n166 = call "总氮报警信息.vi"("data in"=w246) -> ()  [unwired: 11 in]
          }
        }
      }
    }
  }
  n167 = control-ref of="测量模式下拉列表"() -> (w13:refnum<vi>)
  n168 = control-ref of="量程切换阈值"() -> (w11:refnum<vi>)
  n169 = control-ref of="参数下拉列表"() -> (w14:refnum<vi>)
  n170 = control-ref of="量程下拉列表"() -> (w15:refnum<vi>)
  n171 = control-ref of="备用系数"() -> (w10:refnum<vi>)
  n172 = Obtain Queue(name (unnamed)="TN" ("名称（未命名）"), element data type=cluster{"命令":string, "data":variant} {"命令"="", "data"=variant}) -> (queue out=w16:refnum<queue>, error out=w17:errorcluster)  [unwired: 3 in, 1 out]
  n173 = control-ref of="公式"() -> (w12:refnum<vi>)
  n174 = Obtain Notifier(name (unnamed)="TN" ("名称（未命名）"), notification data type=FALSE) -> (notifier out=w1:refnum<notifier>)  [unwired: 2 in, 2 out]
  n175 = while {
    tunnel: w16 -> [w337]
    tunnel: w17 -> [_]
    stop <- FALSE stop-if-true
    w332 = u16 2 items=["总磷"=1, "总氮"=2, "氨氮"=3] ("站号")
    # "试剂填充 172 \n管路清洗108\n氨氮92\n总磷131\n总磷海水147\n总氮76\n总氮海水92"
    n176 = Wait (ms)(milliseconds to wait=u32 1000 ("等待时间（毫秒）")) -> ()  [unwired: 1 out]
    n177 = global read "总氮断电保存全局变量.vi" "流程路径"() -> (w323:path)
    n178 = global read "总氮断电保存全局变量.vi" "VISA Resource"() -> (→"字符串 2":refnum<visa-resource-name>)
    n179 = local write "流程路径"(w323) -> ()
    n180 = Bundle By Name(cluster=cluster{"命令":string, "data":variant} {"命令"="", "data"=variant} ("元素"), "命令"="读状态告警区", "data"=w332) -> (w339:cluster{"命令":string, "data":variant})
    n181 = Bundle By Name(cluster=cluster{"命令":string, "data":variant} {"命令"="", "data"=variant} ("元素"), "命令"="读测量数据区", "data"=w332) -> (w335:cluster{"命令":string, "data":variant})
    n182 = global read "VAR总氮全局变量.vi" "状态告警区"() -> (w324:T4)
    n183 = Unbundle By Name(w324) -> ("系统时间"=w331:timestamp)
    n184 = Enqueue Element(queue=w337, element=w339) -> (queue out=w333:refnum<queue>)  [unwired: 2 in, 2 out]
    n185 = Get Date/Time In Seconds() -> (seconds since 1Jan1904=w330:timestamp)
    n186 = Subtract(x=w330, y=w331) -> (x-y=w329:dbl)
    n187 = Absolute Value(x=w329) -> (abs(x)=w328:dbl)
    n188 = Enqueue Element(queue=w333, element=w335) -> (queue out=w325:refnum<queue>)  [unwired: 2 in, 2 out]
    n189 = Greater Or Equal?(x=w328, y=120.0) -> (x >= y?=w326:bool)
    n190 = case shown="真" w326 {
      tunnel: w325 -> [_ w344]
      frame False {
      }
      frame True {
        n191 = call "总氮启动命令.vi"("参数"=T18 {"站号"=3, "量程切换"=enum."AUTO", "控制命令"=enum."校时", "模式设置"=enum."待机", "测量间隔"=0}) -> ("启动命令"=w343:cluster{"命令":string, "data":variant})  [unwired: 10 in]
        n192 = Enqueue Element(queue=w344, element=w343) -> ()  [unwired: 2 in, 3 out]
      }
    }
  }
  n193 = while {
    tunnel: w16 -> [w353]
    tunnel: w15 -> [w352]
    tunnel: w14 -> [w351]
    tunnel: w13 -> [w350]
    tunnel: w12 -> [w349]
    tunnel: w11 -> [w348]
    tunnel: w10 -> [w347]
    tunnel: w4 -> [_]
    tunnel: w1 -> [w346]
    stop <- FALSE stop-if-true
    n194 = event shown="[9] \"手动启动\": 值改变" {
      selector: _ -> [_ _ _ _ _ _ _ _ _ _ _ _ _ _ _ _ _ _ _ _ _ _]
      dyn-events: _ -> [_ _ _ _ _ _ _ _ _ _ _ _ _ _ _ _ _ _ _ _ _ _]
      timeout: _ -> [_ _ _ _ _ _ _ _ _ _ _ _ _ _ _ _ _ _ _ _ _ _]
      tunnel: w353 -> [_ w364 w390 _ _ _ _ _ _ w457 _ w482 w489 _ _ _ _ _ _ _ _ _]
      tunnel: w352 -> [_ _ _ _ _ _ _ _ _ _ _ _ _ _ _ _ w505 _ w525 w534 _ _]
      tunnel: w351 -> [_ _ _ _ _ _ _ _ _ _ _ _ _ _ _ _ w503 _ w523 w536 w544 w551]
      tunnel: w350 -> [_ _ _ _ _ _ _ _ _ _ _ _ _ _ _ _ w504 _ w524 w535 _ _]
      tunnel: w349 -> [_ _ _ _ _ _ _ _ _ _ _ _ _ _ _ _ w499 _ _ _ _ _]
      tunnel: w348 -> [_ _ _ _ _ _ _ _ _ _ _ _ _ _ _ _ _ _ w519 _ _ _]
      tunnel: w347 -> [_ _ _ _ _ _ _ _ _ _ _ _ _ _ _ _ _ _ _ _ w542 _]
      tunnel: w346 -> [_ _ _ _ _ _ _ _ _ _ _ _ w485 _ _ _ _ _ _ _ _ _]
      event Timeout {
        n195 = event-data() -> ()  [unwired: 1 in, 3 out]
      }
      event "串口设置": Value Change {
        n196 = event-data() -> ()  [unwired: 1 in, 6 out]
        n197 = global read "总氮断电保存全局变量.vi" "MB通信方式选择"() -> (w355:enum16{"串口", "TCP"})
        n198 = global read "总氮断电保存全局变量.vi" "VISA Resource"() -> (w361:refnum<visa-resource-name>)
        n199 = global read "总氮断电保存全局变量.vi" "PORT"() -> (w360:string)
        n200 = global read "总氮断电保存全局变量.vi" "IP"() -> (w356:string)
        n201 = call "串口配置.vi"("PORT"=w360, "IP"=w356, "MB通信方式选择"=w355, "请选择串口:"=w361) -> ("PORT 2"=w358:string, "IP 2"=w359:string, "确认 2"=w362:bool, "VISA资源名称 2"=w363:refnum<visa-resource-name>, "MB通信方式选择 2"=w357:enum16{"串口", "TCP"})  [unwired: 3 in]
        n202 = case shown="真" w362 {
          tunnel: w363 -> [_ w369]
          tunnel: w364 -> [_ w368]
          tunnel: w359 -> [_ w367]
          tunnel: w358 -> [_ w366]
          tunnel: w357 -> [_ w365]
          frame False {
          }
          frame True {
            n203 = flat-sequence {
              tunnel: w369 -> [w373]
              tunnel: w368 -> [w374]
              tunnel: w367 -> [w372]
              tunnel: w366 -> [w371]
              tunnel: w365 -> [w370]
              frame #0 {
                n204 = global write "总氮断电保存全局变量.vi" "IP"(w372) -> ()
                n205 = global write "总氮断电保存全局变量.vi" "PORT"(w371) -> ()
                n206 = global write "总氮断电保存全局变量.vi" "VISA Resource"(w373) -> ()
                n207 = global write "总氮断电保存全局变量.vi" "MB通信方式选择"(w370) -> ()
                n208 = Enqueue Element(queue=w374, element=cluster{"命令":string, "data":variant} {"命令"="启用模块", "data"=variant} ("元素")) -> ()  [unwired: 2 in, 3 out]
              }
              frame #1 {
                n209 = call <vilib>:"Application Directory.vi"() -> ("Application Directory"=w389:path)
                n210 = Build Path(base path=w389, name or relative path="data\\sys.ini" ("名称或相对路径")) -> (appended path=w387:path)
                n211 = call <vilib>:"Open Config Data.vi"("configuration file path"=w387) -> ("error out"=w383:errorcluster, "refnum"=w386:T12)  [unwired: 8 in, 1 out]
                n212 = vi-ref "总氮断电保存全局变量.vi"() -> (w385:refnum<vi>)
                n213 = call <userlib>:"Write Panel to INI__ogtk.vi"("error in (no error)"=w383, "VI ref"=w385, "refnum"=w386) -> ("error out"=w382:errorcluster, "refnum out"=w384:T12)  [unwired: 7 in]
                n214 = call <vilib>:"Close Config Data.vi"("error in (no error)"=w382, "refnum"=w384) -> ("error out"=w377:errorcluster, "file path"=w376:path)  [unwired: 8 in]
                n215 = Open/Create/Replace File(file path (use dialog)=w376, error in=w377) -> (refnum out=w380:refnum<file>, error out=w381:errorcluster)  [unwired: 4 in, 1 out]
                n216 = Flush File(refnum=w380, error in=w381) -> (refnum out=w379:refnum<file>, error out=w378:errorcluster)
                n217 = Close File(refnum=w379, error in=w378) -> ()  [unwired: 2 out]
              }
            }
          }
        }
      }
      event "模块启用": Value Change {
        n218 = event-data() -> ("OldVal"=w391:bool)  [unwired: 1 in, 5 out]
        n219 = case shown="假" w391 {
          tunnel: w390 -> [w392 w394]
          frame False {
            n220 = Enqueue Element(queue=w392, element=cluster{"命令":string, "data":variant} {"命令"="停用模块", "data"=variant} ("元素")) -> ()  [unwired: 2 in, 3 out]
          }
          frame True {
            n221 = Enqueue Element(queue=w394, element=cluster{"命令":string, "data":variant} {"命令"="启用模块", "data"=variant} ("元素")) -> ()  [unwired: 2 in, 3 out]
          }
        }
      }
      event "流程路径": Value Change {
        n222 = event-data() -> ()  [unwired: 1 in, 6 out]
        n223 = flat-sequence {
          frame #0 {
            n224 = local read "流程路径"() -> (w396:path)
            n225 = global write "总氮断电保存全局变量.vi" "流程路径"(w396) -> ()
          }
          frame #1 {
            n226 = call <vilib>:"Application Directory.vi"() -> ("Application Directory"=w410:path)
            n227 = Build Path(base path=w410, name or relative path="data\\sys.ini" ("名称或相对路径")) -> (appended path=w408:path)
            n228 = call <vilib>:"Open Config Data.vi"("configuration file path"=w408) -> ("error out"=w404:errorcluster, "refnum"=w407:T12)  [unwired: 8 in, 1 out]
            n229 = vi-ref "总氮断电保存全局变量.vi"() -> (w406:refnum<vi>)
            n230 = call <userlib>:"Write Panel to INI__ogtk.vi"("error in (no error)"=w404, "VI ref"=w406, "refnum"=w407) -> ("error out"=w403:errorcluster, "refnum out"=w405:T12)  [unwired: 7 in]
            n231 = call <vilib>:"Close Config Data.vi"("error in (no error)"=w403, "refnum"=w405) -> ("error out"=w398:errorcluster, "file path"=w397:path)  [unwired: 8 in]
            n232 = Open/Create/Replace File(file path (use dialog)=w397, error in=w398) -> (refnum out=w401:refnum<file>, error out=w402:errorcluster)  [unwired: 4 in, 1 out]
            n233 = Flush File(refnum=w401, error in=w402) -> (refnum out=w400:refnum<file>, error out=w399:errorcluster)
            n234 = Close File(refnum=w400, error in=w399) -> ()  [unwired: 2 out]
          }
        }
      }
      event "公式一键写入": Value Change {
        n235 = event-data() -> ()  [unwired: 1 in, 6 out]
        n236 = local read "公式"() -> (w411:cluster{"X^2":dbl, "X":dbl, "b":dbl})
        n237 = call "公式复合写入.vi"("公式"=w411) -> ()  [unwired: 11 in]
      }
      event "备用系数一键写入": Value Change {
        n238 = event-data() -> ()  [unwired: 1 in, 6 out]
        n239 = local read "备用系数"() -> (w412:T2)
        n240 = call "量程参数复合参数写入.vi"("备用系数"=w412) -> ()  [unwired: 11 in]
      }
      event "总磷总氮曲线模型": Value Change {
        n241 = event-data() -> ()  [unwired: 1 in, 6 out]
        n242 = local write "公式"("总磷总氮曲线模型") -> ()
      }
      event "质控参数设置": Value Change {
        n243 = event-data() -> ()  [unwired: 1 in, 6 out]
        n244 = global read "总氮断电保存全局变量.vi" "质控参数设置"() -> (w414:T19)
        n245 = call "总氮质控参数设置.vi"("质控参数设置"=w414) -> ("输出簇"=w415:T20)  [unwired: 10 in]
        n246 = Unbundle By Name(w415) -> ("确定"=w416:bool)
        n247 = case shown="真" w416 {
          tunnel: w415 -> [_ w418]
          tunnel: w414 -> [_ w417]
          frame False {
          }
          frame True {
            n248 = flat-sequence {
              tunnel: w418 -> [w425]
              tunnel: w417 -> [w424]
              frame #0 {
                n249 = Unbundle By Name(w425) -> ("跨度值"=w423:dbl, "零点标准液浓度"=w422:dbl, "跨度标准液浓度"=w421:dbl, "标准液标准浓度"=w420:dbl)
                n250 = Bundle By Name(cluster=w424, "跨度值"=w423, "零点标准液浓度"=w422, "跨度标准液浓度"=w421, "标准液标准浓度"=w420) -> (w419:T19)
                n251 = global write "总氮断电保存全局变量.vi" "质控参数设置"(w419) -> ()
              }
              frame #1 {
                n252 = call <vilib>:"Application Directory.vi"() -> ("Application Directory"=w439:path)
                n253 = Build Path(base path=w439, name or relative path="data\\sys.ini" ("名称或相对路径")) -> (appended path=w437:path)
                n254 = call <vilib>:"Open Config Data.vi"("configuration file path"=w437) -> ("error out"=w433:errorcluster, "refnum"=w436:T12)  [unwired: 8 in, 1 out]
                n255 = vi-ref "总氮断电保存全局变量.vi"() -> (w435:refnum<vi>)
                n256 = call <userlib>:"Write Panel to INI__ogtk.vi"("error in (no error)"=w433, "VI ref"=w435, "refnum"=w436) -> ("error out"=w432:errorcluster, "refnum out"=w434:T12)  [unwired: 7 in]
                n257 = call <vilib>:"Close Config Data.vi"("error in (no error)"=w432, "refnum"=w434) -> ("error out"=w427:errorcluster, "file path"=w426:path)  [unwired: 8 in]
                n258 = Open/Create/Replace File(file path (use dialog)=w426, error in=w427) -> (refnum out=w430:refnum<file>, error out=w431:errorcluster)  [unwired: 4 in, 1 out]
                n259 = Flush File(refnum=w430, error in=w431) -> (refnum out=w429:refnum<file>, error out=w428:errorcluster)
                n260 = Close File(refnum=w429, error in=w428) -> ()  [unwired: 2 out]
              }
            }
          }
        }
      }
      event "自动测试量程配置": Value Change {
        n261 = event-data() -> ()  [unwired: 1 in, 6 out]
        n262 = flat-sequence {
          frame #0 {
            n263 = global write "总氮断电保存全局变量.vi" "总氮自动测试量程配置"("自动测试量程配置") -> ()
          }
          frame #1 {
            n264 = call <vilib>:"Application Directory.vi"() -> ("Application Directory"=w454:path)
            n265 = Build Path(base path=w454, name or relative path="data\\sys.ini" ("名称或相对路径")) -> (appended path=w452:path)
            n266 = call <vilib>:"Open Config Data.vi"("configuration file path"=w452) -> ("error out"=w448:errorcluster, "refnum"=w451:T12)  [unwired: 8 in, 1 out]
            n267 = vi-ref "总氮断电保存全局变量.vi"() -> (w450:refnum<vi>)
            n268 = call <userlib>:"Write Panel to INI__ogtk.vi"("error in (no error)"=w448, "VI ref"=w450, "refnum"=w451) -> ("error out"=w447:errorcluster, "refnum out"=w449:T12)  [unwired: 7 in]
            n269 = call <vilib>:"Close Config Data.vi"("error in (no error)"=w447, "refnum"=w449) -> ("error out"=w442:errorcluster, "file path"=w441:path)  [unwired: 8 in]
            n270 = Open/Create/Replace File(file path (use dialog)=w441, error in=w442) -> (refnum out=w445:refnum<file>, error out=w446:errorcluster)  [unwired: 4 in, 1 out]
            n271 = Flush File(refnum=w445, error in=w446) -> (refnum out=w444:refnum<file>, error out=w443:errorcluster)
            n272 = Close File(refnum=w444, error in=w443) -> ()  [unwired: 2 out]
          }
        }
      }
      event "手动启动": Value Change {
        n273 = event-data() -> ()  [unwired: 1 in, 6 out]
        n274 = call "总氮启动参数对话框.vi"() -> ("确认"=w455:bool, "元素"=w456:cluster{"命令":string, "data":variant})  [unwired: 10 in]
        n275 = case shown="真" w455 {
          tunnel: w457 -> [_ w459]
          tunnel: w456 -> [_ w458]
          frame False {
          }
          frame True {
            n276 = Enqueue Element(queue=w459, element=w458) -> ()  [unwired: 2 in, 3 out]
          }
        }
      }
      event "定时启动": Mouse Down {
        n277 = event-data() -> ()  [unwired: 1 in, 6 out]
        n278 = flat-sequence {
          frame #0 {
            n279 = global read "总氮断电保存全局变量.vi" "定时控制"() -> (w461:T5)
            n280 = call "总氮周期设置.vi"("定时控制输入"=w461) -> ("定时控制输出"=w460:T5)  [unwired: 10 in]
            n281 = global write "总氮断电保存全局变量.vi" "定时控制"(w460) -> ()
          }
          frame #1 {
            n282 = call <vilib>:"Application Directory.vi"() -> ("Application Directory"=w475:path)
            n283 = Build Path(base path=w475, name or relative path="data\\sys.ini" ("名称或相对路径")) -> (appended path=w473:path)
            n284 = call <vilib>:"Open Config Data.vi"("configuration file path"=w473) -> ("error out"=w469:errorcluster, "refnum"=w472:T12)  [unwired: 8 in, 1 out]
            n285 = vi-ref "总氮断电保存全局变量.vi"() -> (w471:refnum<vi>)
            n286 = call <userlib>:"Write Panel to INI__ogtk.vi"("error in (no error)"=w469, "VI ref"=w471, "refnum"=w472) -> ("error out"=w468:errorcluster, "refnum out"=w470:T12)  [unwired: 7 in]
            n287 = call <vilib>:"Close Config Data.vi"("error in (no error)"=w468, "refnum"=w470) -> ("error out"=w463:errorcluster, "file path"=w462:path)  [unwired: 8 in]
            n288 = Open/Create/Replace File(file path (use dialog)=w462, error in=w463) -> (refnum out=w466:refnum<file>, error out=w467:errorcluster)  [unwired: 4 in, 1 out]
            n289 = Flush File(refnum=w466, error in=w467) -> (refnum out=w465:refnum<file>, error out=w464:errorcluster)
            n290 = Close File(refnum=w465, error in=w464) -> ()  [unwired: 2 out]
          }
        }
      }
      event "单步测试": Value Change {
        w477 = u16 1 items=["总磷"=1, "氨氮"=3] ("站号")
        n291 = event-data() -> ()  [unwired: 1 in, 6 out]
        n292 = Bundle("站号"=w477, "总磷氨氮调试"="总磷氨氮调试") -> (w476:cluster{"站号":u16, "总磷氨氮调试":u16[]})  [unwired: 1 in]
        n293 = Bundle By Name(cluster=cluster{"命令":string, "data":variant} {"命令"="", "data"=variant} ("元素"), "命令"="debug", "data"=w476) -> (w479:cluster{"命令":string, "data":variant})
        n294 = Enqueue Element(queue=w482, element=w479) -> ()  [unwired: 2 in, 3 out]
      }
      event "停止": Value Change {
        n295 = event-data() -> ()  [unwired: 1 in, 6 out]
        n296 = Enqueue Element(queue=w489, element=cluster{"命令":string, "data":variant} {"命令"="启动", "data"=variant(cluster{"站号":u16, "控制命令输出":u16[]} {"站号"=1, "控制命令输出"=[2816]})} ("元素")) -> (queue out=w486:refnum<queue>)  [unwired: 2 in, 2 out]
        n297 = Cancel Notification(0:w485) -> (8:w484:refnum<notifier>)  [unwired: 1 in, 2 out]
        n298 = Send Notification(notification=TRUE ("通知"), notifier=w484) -> ()  [unwired: 1 in, 2 out]
        n299 = Enqueue Element(queue=w486, element=cluster{"命令":string, "data":variant} {"命令"="启动", "data"=variant(cluster{"站号":u16, "控制命令输出":u16[]} {"站号"=2, "控制命令输出"=[2816]})} ("元素")) -> ()  [unwired: 2 in, 3 out]
      }
      event "设置": Value Change {
        n300 = event-data() -> ()  [unwired: 1 in, 6 out]
        n301 = property on="窗格" class="Pane"("Origin"=T9 {"Horizontal"=0, "Vertical"=628} ("原点")) -> ()  [unwired: 2 in, 2 out]
      }
      event "返回": Value Change {
        n302 = event-data() -> ()  [unwired: 1 in, 6 out]
        n303 = property on="窗格" class="Pane"("Origin"=T9 {"Horizontal"=0, "Vertical"=0} ("原点")) -> ()  [unwired: 2 in, 2 out]
      }
      event "公式.X^2", "公式.X", "公式.b", "量程切换阈值.阈值", "量程切换阈值.标液浓度", "备用系数.量程上限", "备用系数.量程下限", "备用系数.检出限", "备用系数.精度": Mouse Down {
        n304 = event-data() -> ("CtlRef"=w495:refnum<vi>)  [unwired: 1 in, 5 out]
        n305 = property class="DigNum (严格)"(reference=w495) -> (reference out=w493:refnum<vi>, "Value"=w494:dbl)  [unwired: 1 in, 1 out]
        n306 = call "数字键盘.vi"("OldNumber"=w494) -> ("NewNumber"=w492:dbl)
        n307 = property class="DigNum (严格)"(reference=w493, "Val(Sgnl)"=w492) -> ()  [unwired: 1 in, 2 out]
      }
      event "读公式": Value Change {
        n308 = event-data() -> ()  [unwired: 1 in, 6 out]
        n309 = property class="Enum (严格)"(reference=w503) -> ("Value"=w502:enum16{"总磷", "总氮"})  [unwired: 1 in, 2 out]
        n310 = property class="Enum (严格)"(reference=w504) -> ("Value"=w501:enum16{"水样测量", "空白核查", "跨度核查", "标样核查", "加标回收"})  [unwired: 1 in, 2 out]
        n311 = property class="Enum (严格)"(reference=w505) -> ("Value"=w500:enum16{"低量程", "高量程"})  [unwired: 1 in, 2 out]
        n312 = call "总磷总氮公式读取.vi"("量程"=w500, "测量模式"=w501, "测量参数"=w502) -> ("error out"=w497:errorcluster, "公式"=w498:cluster{"X^2":dbl, "X":dbl, "b":dbl})  [unwired: 7 in]
        n313 = property class="Clust (严格)"(reference=w499, "Value"=w498) -> ()  [unwired: 1 in, 2 out]
        n314 = case shown="错误" w497 {
          tunnel: ["读取成功" ("消息") "读取失败" ("消息")] -> w496
          frame No Error {
          }
          frame Error {
          }
        }
        n315 = One Button Dialog(message=w496) -> ()  [unwired: 1 in, 1 out]
      }
      event "写公式": Value Change {
        n316 = event-data() -> ()  [unwired: 1 in, 6 out]
        n317 = call "总磷总氮公式写入.vi"("公式"="公式", "量程"="量程下拉列表", "测量模式"="测量模式下拉列表", "测量参数"="参数下拉列表") -> ("error out"=w510:errorcluster)  [unwired: 7 in]
        n318 = case shown="无错误" w510 {
          tunnel: ["写入成功" ("消息") "写入失败" ("消息")] -> w511
          frame No Error {
          }
          frame Error {
          }
        }
        n319 = One Button Dialog(message=w511) -> ()  [unwired: 1 in, 1 out]
      }
      event "量程切换阈值读取": Value Change {
        n320 = event-data() -> ()  [unwired: 1 in, 6 out]
        n321 = property class="Enum (严格)"(reference=w523) -> ("Value"=w522:enum16{"总磷", "总氮"})  [unwired: 1 in, 2 out]
        n322 = property class="Enum (严格)"(reference=w524) -> ("Value"=w521:enum16{"水样测量", "空白核查", "跨度核查", "标样核查", "加标回收"})  [unwired: 1 in, 2 out]
        n323 = property class="Enum (严格)"(reference=w525) -> ("Value"=w520:enum16{"低量程", "高量程"})  [unwired: 1 in, 2 out]
        n324 = call "总磷总氮量程读取.vi"("量程"=w520, "测量模式"=w521, "测量参数"=w522) -> ("error out"=w516:errorcluster, "量程切换阈值"=w518:cluster{"阈值":dbl, "标液浓度":dbl})  [unwired: 7 in]
        n325 = property class="Clust (严格)"(reference=w519, "Value"=w518) -> ()  [unwired: 1 in, 2 out]
        n326 = case shown="错误" w516 {
          tunnel: ["读取成功" ("消息") "读取失败" ("消息")] -> w517
          frame No Error {
          }
          frame Error {
          }
        }
        n327 = One Button Dialog(message=w517) -> ()  [unwired: 1 in, 1 out]
      }
      event "量程切换阈值写入": Value Change {
        n328 = event-data() -> ()  [unwired: 1 in, 6 out]
        n329 = property class="Enum (严格)"(reference=w536) -> ("Value"=w533:enum16{"总磷", "总氮"})  [unwired: 1 in, 2 out]
        n330 = property class="Enum (严格)"(reference=w535) -> ("Value"=w532:enum16{"水样测量", "空白核查", "跨度核查", "标样核查", "加标回收"})  [unwired: 1 in, 2 out]
        n331 = property class="Enum (严格)"(reference=w534) -> ("Value"=w531:enum16{"低量程", "高量程"})  [unwired: 1 in, 2 out]
        n332 = call "总磷总氮量程写入.vi"("量程切换阈值"="量程切换阈值", "量程"=w531, "测量模式"=w532, "测量参数"=w533) -> ("error out"=w528:errorcluster)  [unwired: 7 in]
        n333 = case shown="无错误" w528 {
          tunnel: ["写入成功" ("消息") "写入失败" ("消息")] -> w529
          frame No Error {
          }
          frame Error {
          }
        }
        n334 = One Button Dialog(message=w529) -> ()  [unwired: 1 in, 1 out]
      }
      event "备用系数读取": Value Change {
        n335 = event-data() -> ()  [unwired: 1 in, 6 out]
        n336 = property class="Enum (严格)"(reference=w544) -> ("Value"=w543:enum16{"总磷", "总氮"})  [unwired: 1 in, 2 out]
        n337 = call "总磷总氮备用系数读取.vi"("测量参数"=w543) -> ("error out"=w539:errorcluster, "备用系数"=w541:T2)  [unwired: 9 in]
        n338 = property class="Clust (严格)"(reference=w542, "Value"=w541) -> ()  [unwired: 1 in, 2 out]
        n339 = case shown="错误" w539 {
          tunnel: ["读取成功" ("消息") "读取失败" ("消息")] -> w540
          frame No Error {
          }
          frame Error {
          }
        }
        n340 = One Button Dialog(message=w540) -> ()  [unwired: 1 in, 1 out]
      }
      event "备用系数写入": Value Change {
        n341 = event-data() -> ()  [unwired: 1 in, 6 out]
        n342 = property class="Enum (严格)"(reference=w551) -> ("Value"=w550:enum16{"总磷", "总氮"})  [unwired: 1 in, 2 out]
        n343 = call "总磷总氮备用系数写入.vi"("备用系数"="备用系数", "测量参数"=w550) -> ("error out"=w547:errorcluster)  [unwired: 9 in]
        n344 = case shown="无错误" w547 {
          tunnel: ["写入成功" ("消息") "写入失败" ("消息")] -> w548
          frame No Error {
          }
          frame Error {
          }
        }
        n345 = One Button Dialog(message=w548) -> ()  [unwired: 1 in, 1 out]
      }
    }
  }
